vi "FFID_Calibration_Purge.vi"   [LabVIEW 2011]
uses:
  ADAM Client/Sub VIs/ADAM Controls/Valco_valve_ph.ctl
types:
  T1 = typedef "Valco_valve_ph.ctl" = u16
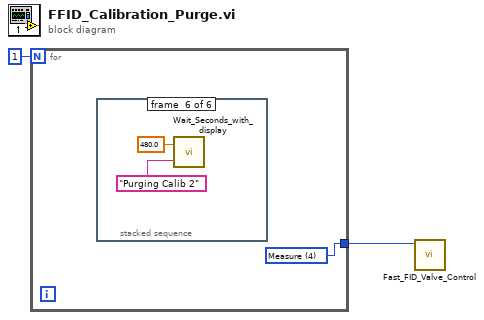
[diagram p0: block diagram]
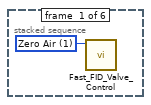
[diagram p2: hidden frame]
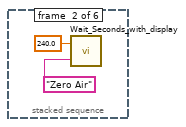
[diagram p3: hidden frame]
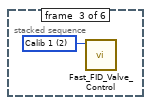
[diagram p4: hidden frame]
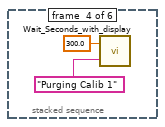
[diagram p5: hidden frame]
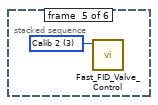
[diagram p6: hidden frame]
diagram:
  n1 = for {
    N: 1 -> [_]
    tunnel: [w3] -> w1
    w3 = T1 4 items=["", "Zero Air", "Calib 1", "Calib 2", "Measure"] ("Requested Position")
    n2 = stacked-sequence {
      frame #0 {
        w4 = T1 1 items=["", "Zero Air", "Calib 1", "Calib 2", "Measure"] ("Requested Position")
        n3 = call "Fast_FID_Valve_Control.vi"("Requested Position"=w4) -> ()  [unwired: 5 in, 2 out]
      }
      frame #1 {
        n4 = call "Wait_Seconds_with_display.vi"("Message"="Zero Air", "Seconds to wait"=240.0) -> ()  [unwired: 1 in, 1 out]
      }
      frame #2 {
        w7 = T1 2 items=["", "Zero Air", "Calib 1", "Calib 2", "Measure"] ("Requested Position")
        n5 = call "Fast_FID_Valve_Control.vi"("Requested Position"=w7) -> ()  [unwired: 5 in, 2 out]
      }
      frame #3 {
        n6 = call "Wait_Seconds_with_display.vi"("Message"="Purging Calib 1", "Seconds to wait"=300.0) -> ()  [unwired: 1 in, 1 out]
      }
      frame #4 {
        w10 = T1 3 items=["", "Zero Air", "Calib 1", "Calib 2", "Measure"] ("Requested Position")
        n7 = call "Fast_FID_Valve_Control.vi"("Requested Position"=w10) -> ()  [unwired: 5 in, 2 out]
      }
      frame #5 {
        n8 = call "Wait_Seconds_with_display.vi"("Message"="Purging Calib 2", "Seconds to wait"=480.0) -> ()  [unwired: 1 in, 1 out]
      }
    }
  }
  n9 = call "Fast_FID_Valve_Control.vi"("Requested Position"=w1) -> ()  [unwired: 5 in, 2 out]
